vi "Construct Channels.vi"(0 "enabled channels":bool[](array[boolean]), 1 "scope":string(combo)) -> (4 "scope":string(combo), 6 "channels":string[](array[string]))   [LabVIEW 2013]
doc: "Constructs an array of channels from the <B>scope</B> and <B>enabled channels</B>. For example, if the <B>enabled channels</B> boolean array has elements 0 and 1 both TRUE with a <B>scope</B> of \"rx\", the resulting <B>enabled channels</B> array will be [\"rx/RF 0\", \"rx/RF 1\"]."
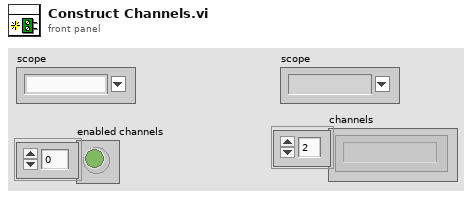
[diagram p1: front panel]
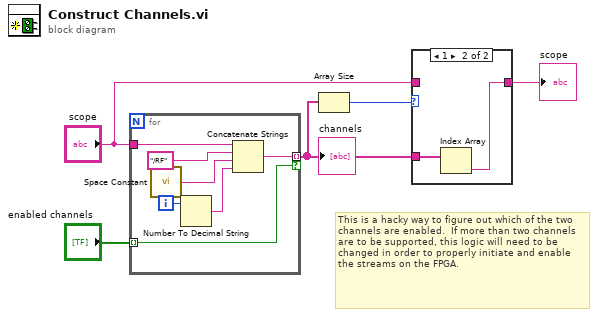
[diagram p0: block diagram]
diagram:
  # "This is a hacky way to figure out which of the two channels are enabled.  If more than two channels are to be supported, this logic will need to be changed in order to properly initiate and enable the streams on the FPGA."
  n1 = for {
    tunnel: "scope" -> [w12]
    tunnel: [w9] -> w3 mode=indexing if=w6
    tunnel: "enabled channels" -> [w6] mode=indexing
    i -> [w10]
    n2 = call <vilib>:"Space Constant.vi"() -> ("String"=w7:string)
    n3 = Number To Decimal String(number=w10) -> (decimal integer string=w11:string)  [unwired: 1 in]
    n4 = Concatenate Strings(w12, "/RF" ("string"), w7, w11) -> (w9:string)
  }
  "channels" <- w3
  n5 = Array Size(array=w3) -> (size(s)=w4:i32)
  n6 = case shown="1" w4 {
    tunnel: w3 -> [_ w15]
    tunnel: [w13 w14] -> w2
    tunnel: "scope" -> [w13 _]
    frame Default {
    }
    frame 1 {
      n7 = Index Array(array=w15) -> (element=w14:string)  [unwired: 1 in]
    }
  }
  "scope" <- w2
